vi "FL_Calculate_phi_theta_etc_for_saving.vi"(0 "Input cluster of data":T1, 1 "Sensor board size":string="Small", 2 "Bridge swap":bool, 3 "Use alternative magnets orientation":bool, 4 "Clamp swap":bool) -> (5 "Output data cluster":T2)   [LabVIEW 2018, in "Tracker.lvlib"]
uses:
  Tracker.lvlib
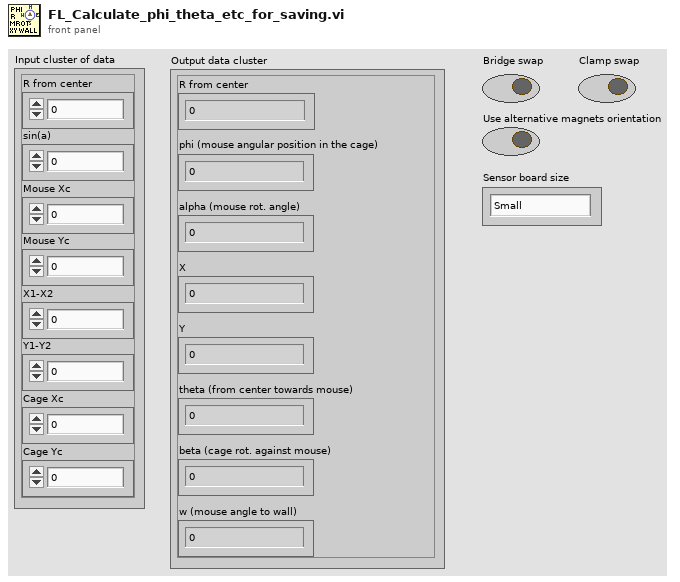
[diagram p1: front panel]
types:
  T1 = cluster{"R from center":dbl, "sin(a)":dbl, "Mouse Xc":dbl, "Mouse Yc":dbl, "X1-X2":dbl, "Y1-Y2":dbl, "Cage Xc":dbl, "Cage Yc":dbl}
  T2 = cluster{"R from center":dbl, "phi (mouse angular position in the cage)":dbl, "alpha (mouse rot. angle)":sgl, "X":dbl, "Y":dbl, "theta (from center towards mouse)":dbl, "beta (cage rot. against mouse)":sgl, "w (mouse angle to wall)":dbl}
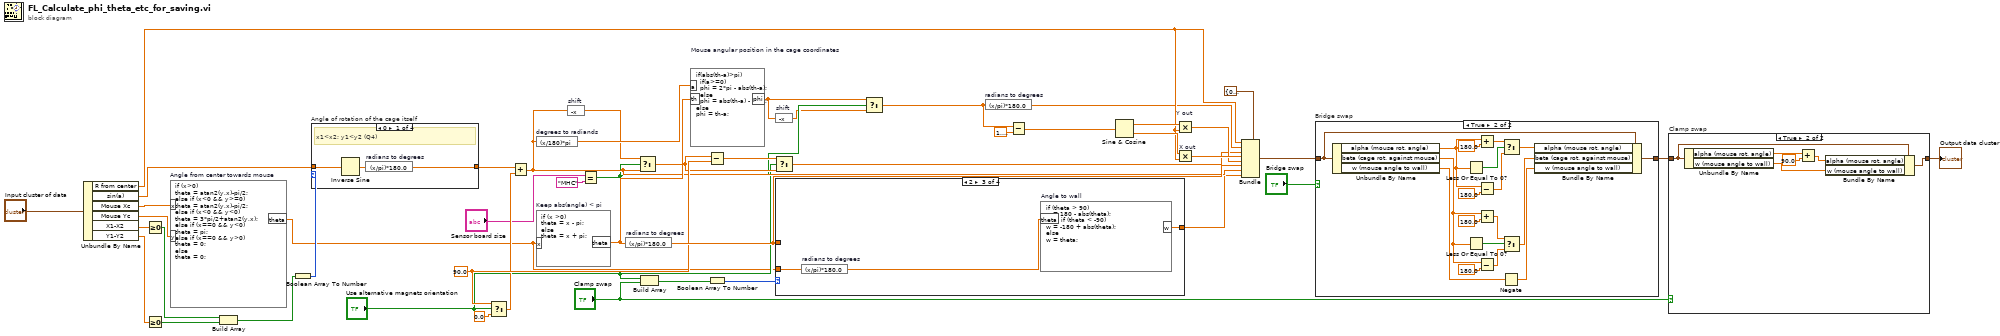
[diagram p0: block diagram]
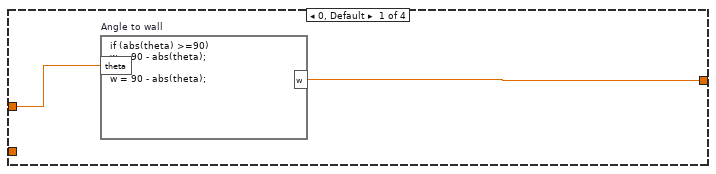
[diagram p3: hidden frame]
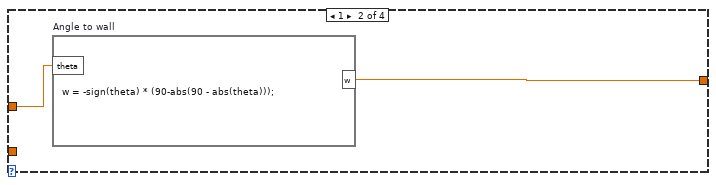
[diagram p4: hidden frame]
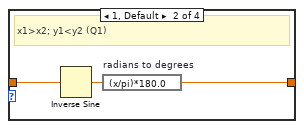
[diagram p7: hidden frame]
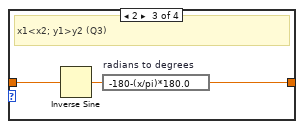
[diagram p8: hidden frame]
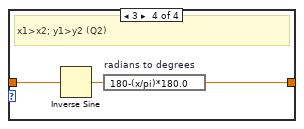
[diagram p9: hidden frame]
diagram:
  w19 = 90.0 ("y")
  n1 = Unbundle By Name("Input cluster of data") -> ("R from center"=w28:dbl, "sin(a)"=w33:dbl, "Mouse Xc"=w32:dbl, "Mouse Yc"=w31:dbl, "X1-X2"=w30:dbl, "Y1-Y2"=w29:dbl)
  n2 = Greater Or Equal To 0?(x=w30) -> (x >= 0?=w47:bool)
  n3 = Greater Or Equal To 0?(x=w29) -> (x >= 0?=w46:bool)
  n4 = formula code="if (x>0)\ntheta = atan2(y,x)-pi/2;\nelse if (x<0 && y>=0)\ntheta = atan2(y,x)-pi/2;\nelse if (x<0 && y<0)\ntheta = 3*pi/2+atan2(y,x);\nelse if (x==0 && y<0)\ntheta = pi;\nelse if (x==0 && y>0)\ntheta = 0;\nelse\ntheta = 0;" "Angle from center towards mouse"("x"=w32, "y"=w31) -> ("theta"=w1:dbl)
  n5 = Build Array(w47, w46) -> (w45:bool[])
  n6 = Boolean Array To Number(Boolean array=w45) -> (number=w44:u32)
  n7 = case "Angle of rotation of the cage itself" shown="0" w44 {
    tunnel: w33 -> [w49 w52 w55 w58]
    tunnel: [w48 w51 w54 w57] -> w22
    frame 0 {
      # "x1<x2; y1<y2 (Q4)"
      n8 = Inverse Sine(1:w49) -> (0:w50:dbl)
      n9 = expression code="(x/pi)*180.0" "radians to degrees"(w50) -> (w48:dbl)
    }
    frame 1, Default {
      # "x1>x2; y1<y2 (Q1)"
      n10 = Inverse Sine(1:w52) -> (0:w53:dbl)
      n11 = expression code="(x/pi)*180.0" "radians to degrees"(w53) -> (w51:dbl)
    }
    frame 2 {
      # "x1<x2; y1>y2 (Q3)"
      n12 = Inverse Sine(1:w55) -> (0:w56:dbl)
      n13 = expression code="-180-(x/pi)*180.0" "radians to degrees"(w56) -> (w54:dbl)
    }
    frame 3 {
      # "x1>x2; y1>y2 (Q2)"
      n14 = Inverse Sine(1:w58) -> (0:w59:dbl)
      n15 = expression code="180-(x/pi)*180.0" "radians to degrees"(w59) -> (w57:dbl)
    }
  }
  n16 = Select(t=w19, s="Use alternative magnets orientation", f=0.0) -> (s? t:f=w18:dbl)
  n17 = Add(x=w22, y=w18) -> (x+y=w14:dbl)
  n18 = expression code="(x/180)*pi" "degrees to radiands"(w14) -> (w40:dbl)
  n19 = formula code="if (x >0)\ntheta = x - pi;\nelse\ntheta = x + pi;" "Keep abs(angle) < pi"("x"=w1) -> ("theta"=w41:dbl)
  n20 = expression code="-x" "shift"(w14) -> (w13:dbl)
  n21 = Equal?(x="Sensor board size", y="MHC") -> (x = y?=w11:bool)
  n22 = expression code="(x/pi)*180.0" "radians to degrees"(w41) -> (w35:dbl)
  n23 = Select(t=w13, s=w11, f=w14) -> (s? t:f=w15:dbl)
  n24 = Build Array("Use alternative magnets orientation", "Clamp swap") -> (w3:bool[])
  n25 = formula code="if(abs(th-a)>pi)\n  if(a>=0)\n  phi = 2*pi - abs(th-a);\n  else\n  phi = abs(th-a) - 2*pi;\nelse\nphi = th-a;" "Mouse angular position in the cage coordinates"("th"=w41, "a"=w40) -> ("phi"=w10:dbl)
  n26 = Subtract(x=w15, y=w19) -> (x-y=w20:dbl)
  n27 = Boolean Array To Number(Boolean array=w3) -> (number=w2:u32)
  n28 = Select(t=w20, s="Use alternative magnets orientation", f=w15) -> (s? t:f=w21:dbl)
  n29 = expression code="-x" "shift"(w10) -> (w9:dbl)
  n30 = case shown="2" w2 {
    tunnel: w35 -> [w61 w63 _ w67]
    tunnel: [w60 w62 w66 w67] -> w6
    tunnel: w1 -> [_ _ w65 _]
    frame 0, Default {
      n31 = formula code="if (abs(theta) >=90)\nw = 90 - abs(theta);\nelse\nw = 90 - abs(theta);" "Angle to wall"("theta"=w61) -> ("w"=w60:dbl)
    }
    frame 1 {
      n32 = formula code="w = -sign(theta) * (90-abs(90 - abs(theta)));" "Angle to wall"("theta"=w63) -> ("w"=w62:dbl)
    }
    frame 2 {
      n33 = expression code="(x/pi)*180.0" "radians to degrees"(w65) -> (w64:dbl)
      n34 = formula code="if (theta > 90)\nw = 180 - abs(theta);\nelse if (theta < -90)\nw = -180 + abs(theta);\nelse\nw = theta;" "Angle to wall"("theta"=w64) -> ("w"=w66:dbl)
    }
    frame 3 {
    }
  }
  n35 = Select(t=w10, s=w11, f=w9) -> (s? t:f=w12:dbl)
  n36 = expression code="(x/pi)*180.0" "radians to degrees"(w12) -> (w27:dbl)
  n37 = Subtract(x=w12, y=1.5707963267948966) -> (x-y=w39:dbl)
  n38 = Sine & Cosine(0:w39) -> (1:w42:dbl, 2:w43:dbl)
  n39 = Multiply "Y out"(x=w42, y=w28) -> (x*y=w36:dbl)
  n40 = Multiply "X out"(x=w43, y=w28) -> (x*y=w37:dbl)
  n41 = Bundle(cluster=T2 {"R from center"=0.0, "phi (mouse angular position in the cage)"=0.0, "alpha (mouse rot. angle)"=0.0, "X"=0.0, "Y"=0.0, "theta (from center towards mouse)"=0.0, "beta (cage rot. against mouse)"=0.0, "w (mouse angle to wall)"=0.0} ("Output data cluster 2"), "R from center"=w28, "phi (mouse angular position in the cage)"=w27, "alpha (mouse rot. angle)"=w21, "X"=w37, "Y"=w36, "theta (from center towards mouse)"=w35, "beta (cage rot. against mouse)"=w14, "w (mouse angle to wall)"=w6) -> (w24:T2)
  n42 = case "Bridge swap" shown="True" "Bridge swap" {
    tunnel: [w68 w80] -> w8
    tunnel: w24 -> [w68 w81]
    frame False {
    }
    frame True {
      n43 = Unbundle By Name(w81) -> ("alpha (mouse rot. angle)"=w79:sgl, "beta (cage rot. against mouse)"=w72:sgl, "w (mouse angle to wall)"=w70:dbl)
      n44 = Less Or Equal To 0?(x=w79) -> (x <= 0?=w86:bool)
      n45 = Less Or Equal To 0?(x=w72) -> (x <= 0?=w73:bool)
      n46 = Add(x=w79, y=sgl 180.0) -> (x+y=w83:sgl)
      n47 = Subtract(x=w79, y=sgl 180.0) -> (x-y=w85:sgl)
      n48 = Add(x=w72, y=sgl 180.0) -> (x+y=w76:sgl)
      n49 = Subtract(x=w72, y=sgl 180.0) -> (x-y=w74:sgl)
      n50 = Negate(x=w70) -> (-x=w69:dbl)
      n51 = Select(t=w83, s=w86, f=w85) -> (s? t:f=w78:sgl)
      n52 = Select(t=w76, s=w73, f=w74) -> (s? t:f=w71:sgl)
      n53 = Bundle By Name(cluster=w81, "alpha (mouse rot. angle)"=w78, "beta (cage rot. against mouse)"=w71, "w (mouse angle to wall)"=w69) -> (w80:T2)
    }
  }
  n54 = case "Clamp swap" shown="True" "Clamp swap" {
    tunnel: [w87 w91] -> w7
    tunnel: w8 -> [w87 w92]
    frame False {
    }
    frame True {
      n55 = Unbundle By Name(w92) -> ("alpha (mouse rot. angle)"=w90:sgl, "w (mouse angle to wall)"=w89:dbl)
      n56 = Add(x=w90, y=sgl 90.0) -> (x+y=w88:sgl)
      n57 = Bundle By Name(cluster=w92, "alpha (mouse rot. angle)"=w88, "w (mouse angle to wall)"=w89) -> (w91:T2)
    }
  }
  "Output data cluster" <- w7
